vi "global_setting.vi"() -> ()   [LabVIEW 2019]
uses:
  Ctrl/agv_config.ctl
  <vilib>/userDefined/High Color/IMAQdx.ctl
  Ctrl/system_hw.ctl
  Ctrl/joystick cfg.ctl
  Ctrl/imu-cfg.ctl
  Ctrl/ledmatrix_data.ctl
panel:
  in  "Settings":T7={"VLP16 cfg"={"h range"={0, 9}, "v range"={0, 9}}, "TIM571 cfg"={"IP"="192.168.0.2", "h range"={0, 9}}, "AGV cfg"={"Port"="COM5", "limits"={"speed limits"={"max"=0.1, "min"=0.0}, "steer limits"={"width"=0.1, "offset"=0.0}}, "dir"=FALSE}, "GPS cfg"={"Port"="COM10", "heading select"="", "PwrPak7_mode select"=[], "rate"=115200}, "PID cfg"={"PID gains"={"proportional gain (Kc)"=0.0025, "integral time (Ti, min)"=0.0, "derivative time (Td, min)"=0.0}, "PID limits"={"output high"=0.05, "output low"=-0.05}, "dt pid"=100}, "Lookahead cfg"={"lookahead pts n"=64.0, "lookahead distance"=5.0}, "Obstacle limit range"={"RL range"=1.1999999999999995, "Point limit"=1}, "State machine parameter"={"angle adjust limit"=20.0}, "waypoint group"={"Waypoint array"=[{"sel"=TRUE, "inv"=FALSE, "path"=path "C:/AGV/Log/0709/refwpt_0709-1 parking-lot to cafe.txt"}, {"sel"=TRUE, "inv"=TRUE, "path"=path "C:/AGV/Log/0709/refwpt_0709-3 hill to cafe.txt"}, {"sel"=TRUE, "inv"=FALSE, "path"=path "C:/AGV/Log/0709/refwpt_0709-3 hill to cafe.txt"}, {"sel"=TRUE, "inv"=TRUE, "path"=path "C:/AGV/Log/0709/refwpt_0709-1 parking-lot to cafe.txt"}]}, "State machine cfg"={" turn angular speed"=0.5, "move linear speed"=0.5, "decrease factor linear speed"=80.0, "adjust angle margin"=9.0}, "camera cfg"={"Port"="cam2", "Camera file"=path "C:/AGV/Config/camera/C920.icd"}, "ROI-clamp"={"Global Rectangle"=[], "Contours"=[]}, "x-center"=0.0, "Image Size"={"x"=0, "y"=0}, "Angle deg"=0.0, "Vison cfg"={"Clamp Settings"={"Contrast"=44, "Filter width"=8, "Steepness"=8, "Subsampling Ratio"=12, "Show Search Area"=TRUE, "Show Search Lines"=TRUE, "Show Edges Found"=TRUE, "Show Result"=TRUE}, "Range"={"Lower value"=128.0, "Upper value"=255.0}, "N of Erosion 1"=2, "N of Erosion 2"=2}, "RPLidar cfg"={"port"="COM6", "dt"=6, "update"=8, "speed"=272, "rate "=256000}, "HW info"={"AGV"=enum."ERP42", "Lidar 1"=enum."none", "Lidar 2"=enum."none", "GPS"=enum."none", "Camera"=enum."none", "Joystick"=enum."none", "sound"=enum."none", "IMU"=enum."none", "Led"=enum."none"}, "Joystick cfg"={"Type"=enum."Logitech F710", "steer limit"={"min"=10.0, "max"=42.0, "scale"=0.0, "offset"=0.0}, "speed limit"={"min"=10.0, "max"=42.0, "pwm max"=0.0}, "ID"=0, "joystick max"=0.0}, "IMU cfg"={"Port"="COM10", "offset"=0.0, "rate"=115200}, "ledmatrix cfg"={"ip"="", "data"="", "Port"="COM6", "time"=""}} {"RPLidar cfg"."speed" scale=100.0..1000.0; "Vison cfg"."Range"."Upper value" scale=0.0..255.0; "Vison cfg"."Range"."Lower value" scale=0.0..255.0; "PID cfg"."PID limits"."output low" format="%.2f"; "PID cfg"."PID limits"."output high" format="%.2f"; "PID cfg"."PID gains"."derivative time (Td, min)" format="%.6f"; "PID cfg"."PID gains"."integral time (Ti, min)" format="%.6f"; "PID cfg"."PID gains"."proportional gain (Kc)" format="%.6f"; "TIM571 cfg"."h range" scale=-180.0..180.0; "VLP16 cfg"."v range" scale=-15.0..15.0; "VLP16 cfg"."h range" scale=-180.0..180.0}
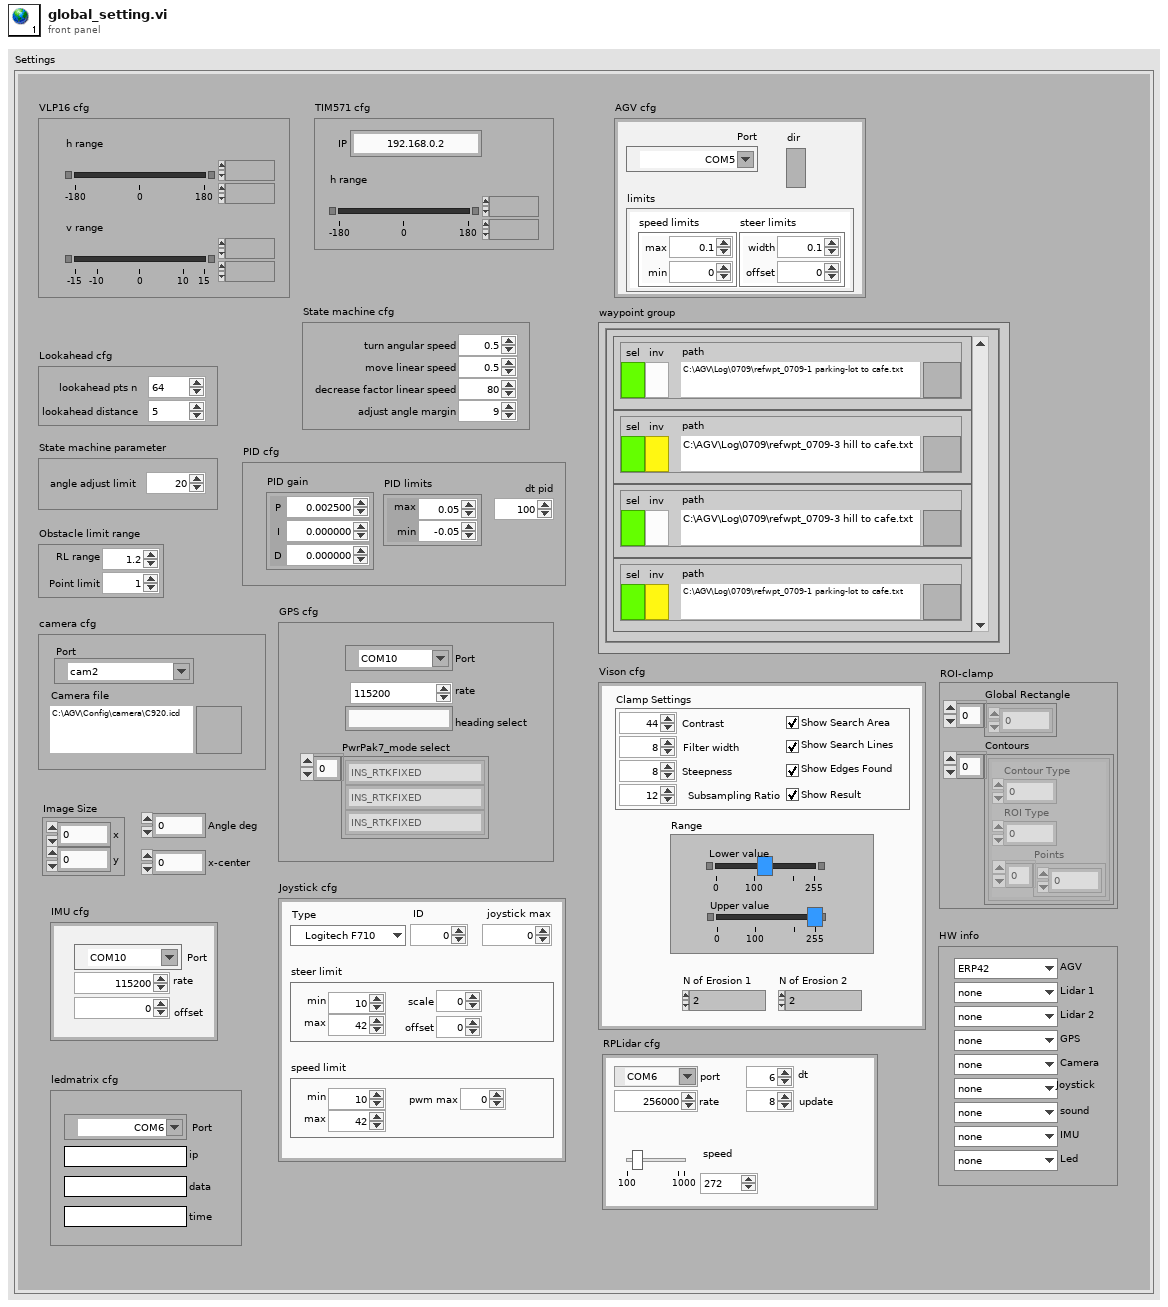
[diagram p1: front panel]
types:
  T1 = typedef "agv_config.ctl" = cluster{"Port":refnum<visa-resource-name>, "limits":cluster{"speed limits":cluster{"max":dbl, "min":dbl}, "steer limits":cluster{"width":dbl, "offset":dbl}}, "dir":bool}
  T2 = typedef "IMAQdx.ctl" = refnum<k21>
  T3 = typedef "system_hw.ctl" = cluster{"AGV":enum16{"none", "ERP42", "Scout", "SBC", "ASV"}, "Lidar 1":enum16{"none", "VLP16", "TIM571", "RPLidar A2", "RPLidar A3"}, "Lidar 2":enum16{"none", "VLP16", "TIM571", "RPLidar A2", "RPLidar A3"}, "GPS":enum16{"none", "F9P", "M8P", "PwrPak7", "19X HVS"}, "Camera":enum16{"none", "C920", "C922", "GT1290C", "MS LifeCam"}, "Joystick":enum16{"none", "joystick"}, "sound":enum16{"none", "speaker"}, "IMU":enum16{"none", "MW-AHRSv1"}, "Led":enum16{"none", "LedMatrix 8x32"}}
  T4 = typedef "joystick cfg.ctl" = cluster{"Type":enum16{"Logitech F710", "Xbox"}, "steer limit":cluster{"min":dbl, "max":dbl, "scale":dbl, "offset":dbl}, "speed limit":cluster{"min":dbl, "max":dbl, "pwm max":dbl}, "ID":i32, "joystick max":dbl}
  T5 = typedef "imu-cfg.ctl" = cluster{"Port":refnum<visa-resource-name>, "offset":dbl, "rate":u32}
  T6 = typedef "ledmatrix_data.ctl" = cluster{"ip":string, "data":string, "Port":refnum<visa-resource-name>, "time":string}
  T7 = cluster{"VLP16 cfg":cluster{"h range":cluster{i16, i16}, "v range":cluster{i8, i8}}, "TIM571 cfg":cluster{"IP":string, "h range":cluster{i16, i16}}, "AGV cfg":T1, "GPS cfg":cluster{"Port":refnum<visa-resource-name>, "heading select":string, "PwrPak7_mode select":string[], "rate":u32}, "PID cfg":cluster{"PID gains":cluster{"proportional gain (Kc)":dbl, "integral time (Ti, min)":dbl, "derivative time (Td, min)":dbl}, "PID limits":cluster{"output high":dbl, "output low":dbl}, "dt pid":u32}, "Lookahead cfg":cluster{"lookahead pts n":dbl, "lookahead distance":dbl}, "Obstacle limit range":cluster{"RL range":dbl, "Point limit":u16}, "State machine parameter":cluster{"angle adjust limit":dbl}, "waypoint group":cluster{"Waypoint array":cluster{"sel":bool, "inv":bool, "path":path}[]}, "State machine cfg":cluster{" turn angular speed":dbl, "move linear speed":dbl, "decrease factor linear speed":dbl, "adjust angle margin":dbl}, "camera cfg":cluster{"Port":T2, "Camera file":path}, "ROI-clamp":cluster{"Global Rectangle":i32[], "Contours":cluster{"Contour Type":u32, "ROI Type":u32, "Points":i32[]}[]}, "x-center":dbl, "Image Size":cluster{"x":i32, "y":i32}, "Angle deg":sgl, "Vison cfg":cluster{"Clamp Settings":cluster{"Contrast":i32, "Filter width":i32, "Steepness":i32, "Subsampling Ratio":u32, "Show Search Area":bool, "Show Search Lines":bool, "Show Edges Found":bool, "Show Result":bool}, "Range":cluster{"Lower value":sgl, "Upper value":sgl}, "N of Erosion 1":i32, "N of Erosion 2":i32}, "RPLidar cfg":cluster{"port":refnum<visa-resource-name>, "dt":u32, "update":u8, "speed":u16, "rate ":u32}, "HW info":T3, "Joystick cfg":T4, "IMU cfg":T5, "ledmatrix cfg":T6}
diagram:
